vi "getData_v5_2FIFO.vi"() -> ()   [LabVIEW 2014]
uses:
  <vilib>/rvi/interface/nirviOpenFPGA/nirviOpenFPGA.xnode
  <vilib>/rvi/interface/nirviCloseFPGA/nirviCloseFPGA.xnode
  <vilib>/Utility/file.llb/Write To Spreadsheet File (DBL).vi
  <vilib>/rvi/interface/nirviMethod/nirviMethod.xnode
  FPGA Bitfiles/test0304_FPGATarget_imptestv4_skixW0YTJzY.lvbitx
  FPGA VIs/imp_test_v4.vi
  <vilib>/FPGAPlugInAG/cRIO-9039/niLvFpga_Close_cRIO-9039.vi
  <vilib>/FPGAPlugInAG/cRIO-9039/niLvFpga_ReadFifo_cRIO-9039.vi
  <vilib>/rvi/errors/niLvFpgaMergeErrorWithErrorCode.vi
  <vilib>/FPGAPlugInAG/cRIO-9039/niLvFpga_Open_cRIO-9039.vi
panel:
  out "Elements Remaining_y":u32=10000
  out "FIFO_y empty":bool
  out "Timer (Sec)":u32
  out "FIFO_p empty":bool
  out "Elements Remaining_p":u32=10000
  in  "Time_read":i32=10000
  out "message":string=" INSTRUCTIONS:\r\rNormal Use:  When using subVIs that incorporate the error in/error out (or error I/O) structure, place this handler where you want to inform the user of an error, typically at the end of the I/O data path, as the last action of the program.  If the error in error? is ERROR, the handler creates a message describing the error and its source.  If the type of dialog = 1 (default), the message is displayed to the user, who can only acknowedge it.  If the type = 2, the user can acknowledge the message or abort execution; aborting a program with active I/O is not recommended.  If the type = 0, no message is displayed; this is used to process the error programmatically, and the error out cluster elements are wired to individual terminals for that reason.  \r\rOther Use:\n\r\nlocal testing.  To test the error code of a subVI or function that does not have the error I/O structure, you can wire its error code and a source string to the local error code and error source inputs.  If error in error? indicates no error and error code is not equal to 0, the local code and source are substituted for the error in values, and error? is set TRUE (ERROR)."
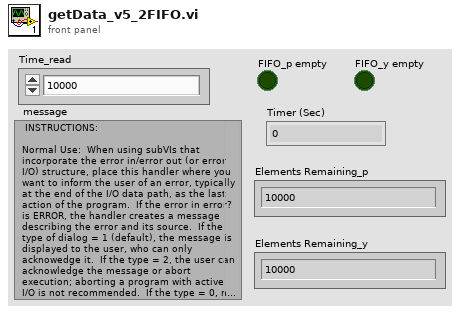
[diagram p1: front panel]
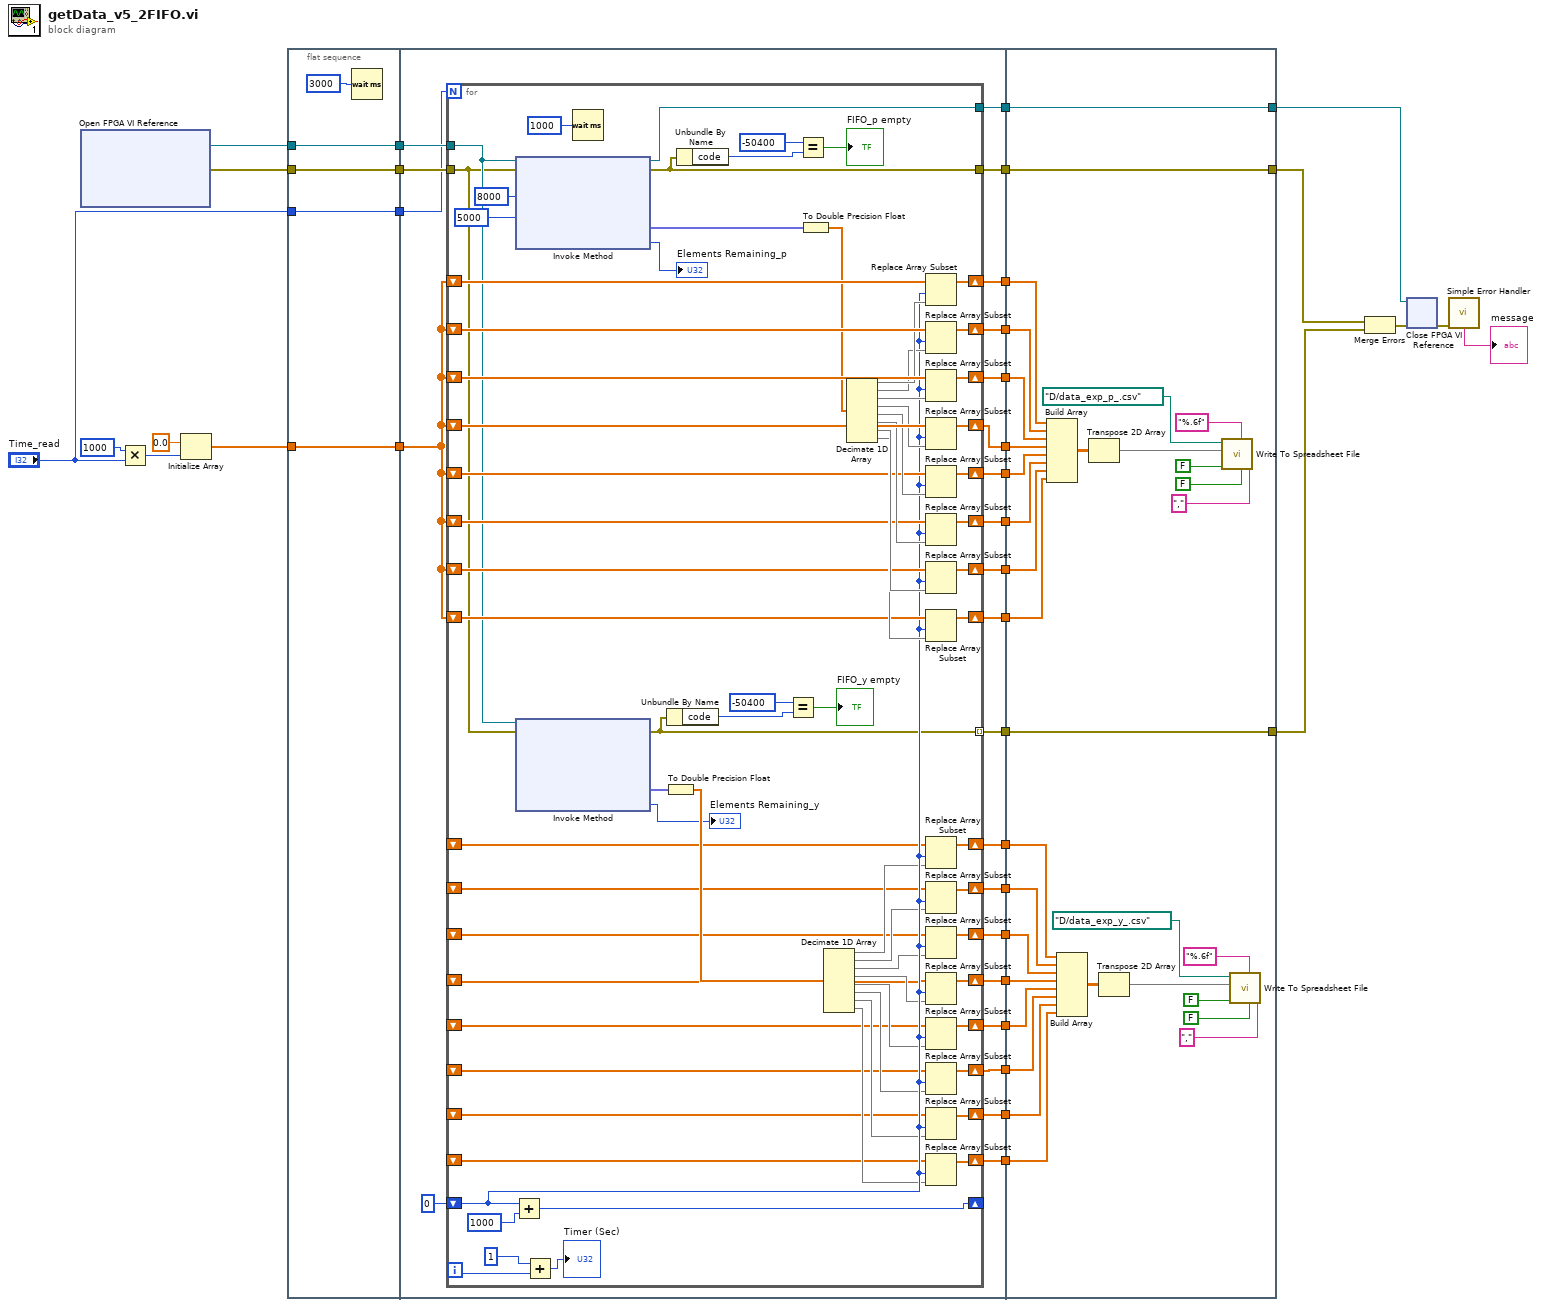
[diagram p0: block diagram]
diagram:
  n1 = xnode "Open FPGA VI Reference"() -> ("FPGA VI Reference Out"=w14:refnum<k20>, "error out"=w15:errorcluster)  [unwired: 2 in]
  n2 = Multiply(x=1000 ("y"), y="Time_read") -> (x*y=w31:i32)
  n3 = Initialize Array(0.0 ("element"), w31) -> (w33:dbl[])
  n4 = flat-sequence {
    tunnel: "Time_read" -> [w38]
    tunnel: w15 -> [w39]
    tunnel: w14 -> [w40]
    tunnel: w33 -> [w41]
    tunnel: [w41] -> w19
    tunnel: [w40] -> w18
    tunnel: [w39] -> w17
    tunnel: [w38] -> w16
    tunnel: [w62] -> w29
    tunnel: [w61] -> w28
    tunnel: [w60] -> w27
    tunnel: [w59] -> w26
    tunnel: [w58] -> w25
    tunnel: [w56] -> w24
    tunnel: [w55] -> w23
    tunnel: [w54] -> w22
    tunnel: [w53] -> w21
    tunnel: [w52] -> w20
    tunnel: w19 -> [w57]
    tunnel: w18 -> [w64]
    tunnel: w17 -> [w63]
    tunnel: w16 -> [w51]
    tunnel: [w50] -> w13
    tunnel: [w49] -> w12
    tunnel: [w48] -> w11
    tunnel: [w47] -> w10
    tunnel: [w46] -> w9
    tunnel: [w45] -> w8
    tunnel: [w44] -> w7
    tunnel: [w43] -> w6
    tunnel: [w42] -> w5
    tunnel: w29 -> [w169]
    tunnel: w28 -> [w168]
    tunnel: w27 -> [w167]
    tunnel: [w172] -> w1
    tunnel: w26 -> [w172]
    tunnel: [w171] -> w4
    tunnel: w25 -> [w171]
    tunnel: w24 -> [w166]
    tunnel: w23 -> [w165]
    tunnel: w22 -> [w163]
    tunnel: w21 -> [w164]
    tunnel: w20 -> [w170]
    tunnel: [w155] -> w3
    tunnel: w13 -> [w155]
    tunnel: w12 -> [w154]
    tunnel: w11 -> [w153]
    tunnel: w10 -> [w152]
    tunnel: w9 -> [w151]
    tunnel: w8 -> [w150]
    tunnel: w7 -> [w149]
    tunnel: w6 -> [w148]
    tunnel: w5 -> [w147]
    frame #0 {
      n5 = Wait (ms)(milliseconds to wait=u32 3000 ("y")) -> ()  [unwired: 1 out]
    }
    frame #1 {
      n6 = for {
        N: w51 -> [_]
        shift-right: [w137] -> _
        shift-left: 0 -> [w99]
        shift-right: [w126] -> w62
        shift-left: w57 -> [w135]
        shift-right: [w125] -> w61
        shift-left: w57 -> [w134]
        shift-right: [w124] -> w60
        shift-left: w57 -> [w133]
        shift-right: [w127] -> w52
        shift-left: w57 -> [w136]
        tunnel: w64 -> [w98]
        tunnel: w63 -> [w97]
        tunnel: [w105] -> w59
        tunnel: [w106] -> w58
        shift-right: [w118] -> w56
        shift-left: w57 -> [w119]
        shift-right: [w116] -> w55
        shift-left: w57 -> [w117]
        shift-right: [w115] -> w53
        shift-left: w57 -> [w114]
        shift-right: [w112] -> w54
        shift-left: w57 -> [w113]
        tunnel: [w93] -> w50 mode=indexing
        shift-right: [w75] -> w49
        shift-left: _ -> [w74]
        shift-right: [w76] -> w48
        shift-left: _ -> [w73]
        shift-right: [w77] -> w47
        shift-left: _ -> [w72]
        shift-right: [w78] -> w46
        shift-left: _ -> [w71]
        shift-right: [w79] -> w45
        shift-left: _ -> [w70]
        shift-right: [w80] -> w44
        shift-left: _ -> [w69]
        shift-right: [w81] -> w43
        shift-left: _ -> [w68]
        shift-right: [w82] -> w42
        shift-left: _ -> [w67]
        i -> [w102]
        n7 = Add(x=w99, y=1000) -> (x+y=w137:i32)
        n8 = xnode "Invoke Method"("FPGA VI Reference In"=w98, "error in"=w97, "Number of Elements"=u32 8000, "Timeout (ms)"=5000) -> ("FPGA VI Reference Out"=w105:refnum<k20>, "error out"=w106:errorcluster, "Data"=w103:fxp<+/-,42,20>[], "Elements Remaining"=→"Elements Remaining_p":u32)
        n9 = xnode "Invoke Method"("FPGA VI Reference In"=w98, "error in"=w97) -> ("error out"=w93:errorcluster, "Data"=w91:fxp<+/-,42,20>[], "Elements Remaining"=→"Elements Remaining_y":u32)  [unwired: 2 in, 1 out]
        n10 = Add(x=1, y=w102) -> (x+y=→"Timer (Sec)":i32)
        n11 = Wait (ms)(milliseconds to wait=u32 1000 ("y")) -> ()  [unwired: 1 out]
        n12 = To Double Precision Float(number=w91) -> (double precision float=w92:dbl[])
        n13 = Unbundle By Name(w93) -> ("code"=w95:i32)
        n14 = Unbundle By Name(w106) -> ("code"=w110:i32)
        n15 = Equal?(x=-50400 ("y"), y=w95) -> (x = y?=→"FIFO_y empty":bool)
        n16 = Equal?(x=-50400 ("y"), y=w110) -> (x = y?=→"FIFO_p empty":bool)
        n17 = To Double Precision Float(number=w103) -> (double precision float=w132:dbl[])
        n18 = Decimate 1D Array(w92) -> (w90:dbl[], w89:dbl[], w88:dbl[], w87:dbl[], w86:dbl[], w85:dbl[], w84:dbl[], w83:dbl[])
        n19 = Decimate 1D Array(w132) -> (w131:dbl[], w130:dbl[], w129:dbl[], w128:dbl[], w123:dbl[], w122:dbl[], w121:dbl[], w120:dbl[])
        n20 = Replace Array Subset(array=w136, new element=w131, index=w99) -> (w127:dbl[])
        n21 = Replace Array Subset(array=w135, new element=w130, index=w99) -> (w126:dbl[])
        n22 = Replace Array Subset(array=w134, new element=w129, index=w99) -> (w125:dbl[])
        n23 = Replace Array Subset(array=w133, new element=w128, index=w99) -> (w124:dbl[])
        n24 = Replace Array Subset(array=w119, new element=w123, index=w99) -> (w118:dbl[])
        n25 = Replace Array Subset(array=w117, new element=w122, index=w99) -> (w116:dbl[])
        n26 = Replace Array Subset(array=w114, new element=w121, index=w99) -> (w115:dbl[])
        n27 = Replace Array Subset(array=w113, new element=w120, index=w99) -> (w112:dbl[])
        n28 = Replace Array Subset(array=w74, new element=w90, index=w99) -> (w75:dbl[])
        n29 = Replace Array Subset(array=w73, new element=w89, index=w99) -> (w76:dbl[])
        n30 = Replace Array Subset(array=w72, new element=w88, index=w99) -> (w77:dbl[])
        n31 = Replace Array Subset(array=w71, new element=w87, index=w99) -> (w78:dbl[])
        n32 = Replace Array Subset(array=w70, new element=w86, index=w99) -> (w79:dbl[])
        n33 = Replace Array Subset(array=w69, new element=w85, index=w99) -> (w80:dbl[])
        n34 = Replace Array Subset(array=w68, new element=w84, index=w99) -> (w81:dbl[])
        n35 = Replace Array Subset(array=w67, new element=w83, index=w99) -> (w82:dbl[])
      }
    }
    frame #2 {
      n36 = Build Array(w170, w169, w168, w167, w166, w165, w164, w163) -> (w156:dbl[][])
      n37 = Build Array(w154, w153, w152, w151, w150, w149, w148, w147) -> (w146:dbl[][])
      n38 = Transpose 2D Array(2D array=w156) -> (transposed array=w161:dbl[][])
      n39 = Transpose 2D Array(2D array=w146) -> (transposed array=w141:dbl[][])
      n40 = call-poly <vilib>:"Write To Spreadsheet File.vi"("delimiter (\\t)"="," ("delimiter (\\t)"), "transpose? (no:F)"=FALSE, "format (%.3f)"="%.6f" ("format (%d)"), "append to file? (new file:F)"=FALSE, "2D data"=w161, "file path (dialog if empty)"=path "D:/data_exp_p_.csv") -> ()  [unwired: 2 in, 1 out]
      n41 = call-poly <vilib>:"Write To Spreadsheet File.vi"("delimiter (\\t)"="," ("delimiter (\\t)"), "transpose? (no:F)"=FALSE, "format (%.3f)"="%.6f" ("format (%d)"), "append to file? (new file:F)"=FALSE, "2D data"=w141, "file path (dialog if empty)"=path "D:/data_exp_y_.csv") -> ()  [unwired: 2 in, 1 out]
    }
  }
  n42 = Merge Errors(w4, w3) -> (w2:errorcluster)
  n43 = xnode "Close FPGA VI Reference"("FPGA VI Reference In"=w1, "error in"=w2) -> ("error out"=w35:errorcluster)
  n44 = call <vilib>:"Simple Error Handler.vi"("error in (no error)"=w35) -> ("message"=→"message":string)  [unwired: 4 in, 4 out]
